vi "TDS Comms Connect.vi"(8 "error in (no error)":errorcluster, 10 "Connection Parameters":string, 11 "Address":string) -> (0 "error out":errorcluster)   [LabVIEW 2025, in "Interface Functions.lvlib"]
uses:
  Interface Functions.lvlib
panel:
  # "Comms Connect"
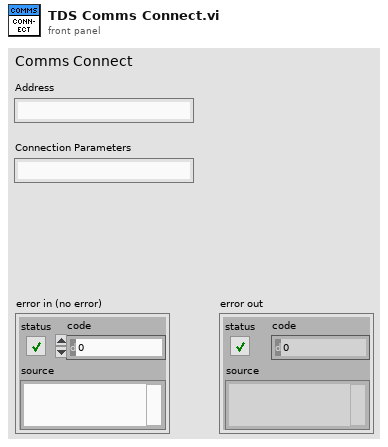
[diagram p1: front panel]
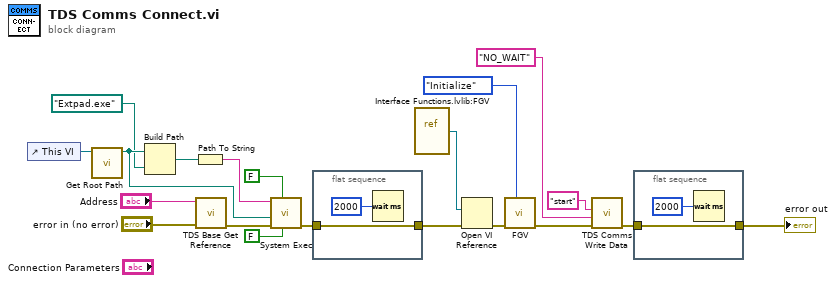
[diagram p0: block diagram]
diagram:
  n1 = control-ref of="This VI"() -> (w5:refnum<vi>)
  n2 = call "Get Root Path.vi"("VI in"=w5) -> ("Extpad Directory"=w16:path)  [unwired: 10 in]
  n3 = Build Path(base path=w16, name or relative path=path "Extpad.exe") -> (appended path=w4:path)
  n4 = Path To String(path=w4) -> (string=w17:string)
  n5 = call "TDS Base Get Reference.vi"("error in (no error)"="error in (no error)", "Address"="Address") -> ("error out"=w18:errorcluster)  [unwired: 8 in, 1 out]
  n6 = call <vilib>:"System Exec.vi"("run minimized? (F)"=FALSE, "wait until completion? (T)"=FALSE, "error in (no error)"=w18, "working directory"=w16, "command line"=w17) -> ("error out"=w14:errorcluster)  [unwired: 3 in, 3 out]
  n7 = flat-sequence {
    tunnel: [w21] -> w10
    tunnel: w14 -> [w21]
    frame #0 {
      n8 = Wait (ms)(milliseconds to wait=u32 2000) -> ()  [unwired: 1 out]
    }
  }
  n9 = vi-ref "Interface Functions.lvlib:FGV.vi"() -> (w9:refnum<vi>)
  n10 = Open VI Reference(vi path=w9, error in (no error)=w10) -> (error out=w8:errorcluster)  [unwired: 4 in, 1 out]
  n11 = call "FGV.vi"("Action"=enum16{"Initialize", "Read", "Write"}."Initialize", "error in (no error)"=w8) -> ("error out"=w6:errorcluster)  [unwired: 7 in, 2 out]
  n12 = call "TDS Comms Write Data.vi"("error in (no error)"=w6, "Write Settings"="NO_WAIT", "Write Data"="start") -> ("error out"=w11:errorcluster)  [unwired: 7 in, 1 out]
  n13 = flat-sequence {
    tunnel: [w23] -> w1
    tunnel: w11 -> [w23]
    frame #0 {
      n14 = Wait (ms)(milliseconds to wait=u32 2000) -> ()  [unwired: 1 out]
    }
  }
  "error out" <- w1
